vi "DisableEnable Download Button.vi"(8 "error in (no error)":errorcluster, 11 "Disable?":bool) -> (0 "error out":errorcluster)   [LabVIEW 2010, in "CAN Log Transfer and Convert.lvlib"]
uses:
  CAN Log Transfer and Convert.lvlib
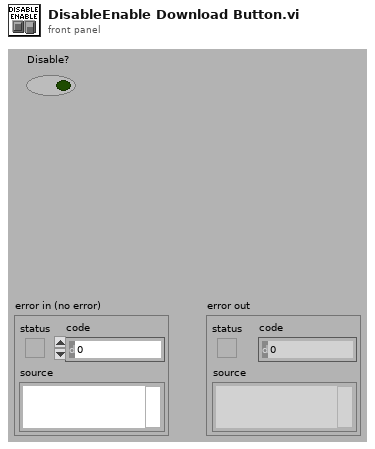
[diagram p1: front panel]
types:
  T1 = enum8{"Enabled", "Disabled", "Disabled and Grayed Out"}
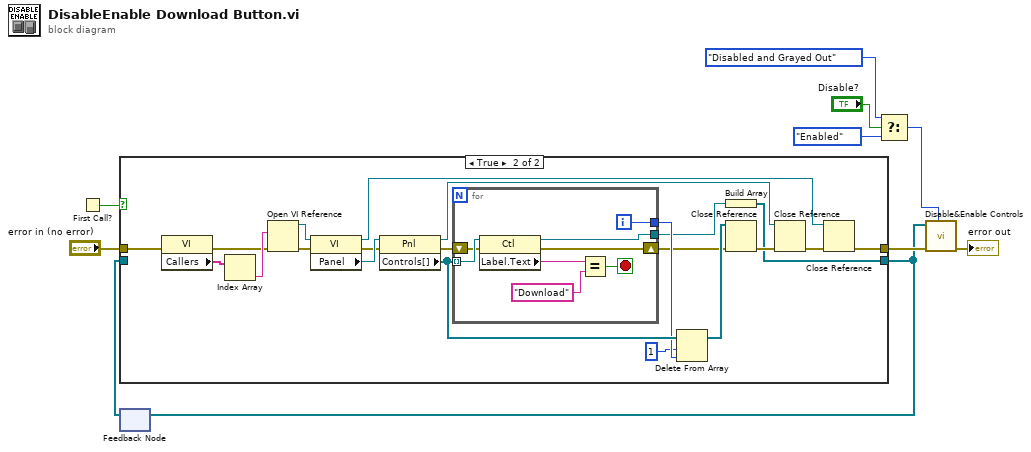
[diagram p0: block diagram]
diagram:
  n1 = First Call?() -> (First Call?: T/F=w9:bool)
  n2 = feedback #1() -> (w8:refnum<vi>[])  [unwired: 1 in]
  n3 = case shown="True" w9 {
    tunnel: "error in (no error)" -> [w11 w33]
    tunnel: [w12 w13] -> w6
    tunnel: w8 -> [w12 _]
    tunnel: [w11 w14] -> w7
    frame False {
    }
    frame True {
      n4 = property class="VI"(error in=w33) -> (error out=w30:errorcluster, "Callers"=w32:string[])  [unwired: 1 in, 1 out]
      n5 = Index Array(array=w32) -> (element=w31:string)  [unwired: 1 in]
      n6 = Open VI Reference(vi path=w31, error in (no error)=w30) -> (vi reference=w29:refnum<vi>, error out=w28:errorcluster)  [unwired: 4 in]
      n7 = property class="VI"(reference=w29, error in=w28) -> (reference out=w16:refnum<vi>, error out=w18:errorcluster, "Panel"=w27:refnum<vi>)
      n8 = property class="Pnl"(reference=w27, error in=w18) -> (reference out=w19:refnum<vi>, error out=w26:errorcluster, "Controls[]"=w25:refnum<vi>[])
      n9 = for {
        tunnel: w25 -> [w41] mode=indexing
        tunnel: [w37] -> w15
        shift-right: [w35] -> w22
        shift-left: w26 -> [w36]
        tunnel: [w34] -> w24
        i -> [w34]
        stop <- w38 stop-if-true
        n10 = property class="Ctl"(reference=w41, error in=w36) -> (reference out=w37:refnum<vi>, error out=w35:errorcluster, "Label.Text"=w40:string)
        n11 = Equal?(x=w40, y="Download") -> (x = y?=w38:bool)
      }
      n12 = Delete From Array(array=w25, length=1, index=w24) -> (array with subset deleted=w23:refnum<vi>[])  [unwired: 1 out]
      n13 = Build Array(w15) -> (w13:refnum<vi>[])
      n14 = Close Reference(reference=w23, error in (no error)=w22) -> (error out=w20:errorcluster)
      n15 = Close Reference(reference=w19, error in (no error)=w20) -> (error out=w17:errorcluster)
      n16 = Close Reference(reference=w16, error in (no error)=w17) -> (error out=w14:errorcluster)
    }
  }
  n17 = feedback-in #1(w6) -> ()
  n18 = Select(t=T1."Disabled and Grayed Out", s="Disable?", f=T1."Enabled" ("State")) -> (s? t:f=w3:T1)
  n19 = call "Disable&Enable Controls.vi"("State"=w3, "error in (no error)"=w7, "Controls"=w6) -> ("error out"=→"error out":errorcluster)  [unwired: 8 in]
